vi "ResonanceScanner_V2.vi"() -> ()   [LabVIEW 2012]
uses:
  <vilib>/Platform/TimedLoop/XDataNode/timing_clust.ctl
  <vilib>/Platform/TimedLoop/XDataNode/nitl_modes.ctl
  <vilib>/Platform/TimedLoop/XDataNode/wakeup.ctl
  <vilib>/rvi/eio/common/nirviEmuTemplateMethod_errors.vi
  <vilib>/rvi/FIFO/Fifo_Resource/nirvififoEmulationSetSize.vi
  <vilib>/rvi/DataTransferAndStorage/Container/Common/niFpgaContainerGetUniqueNameForEmu.vi
  <vilib>/rvi/Emulation/niFpgaSctlEmulationRegisterWithScheduler.vi
  <vilib>/rvi/errors/niFpgaSetErrorForExecOnDevCompSimple.vi
  <vilib>/rvi/eio/common/nirviEmuReportErrorAndStop.vi
  <vilib>/rvi/Emulation/niFpgaSctlEmulationFifoFullMgr.vi
  <vilib>/rvi/Emulation/niFpgaSctlEmulationResourceMgr.vi
  <vilib>/rvi/Emulation/niFpgaSctlEmulationScheduler.vi
  <vilib>/rvi/interface/RandomDataEmulation/nirviRandomDataFPGAFIFO.vi
  <vilib>/rvi/interface/RandomDataEmulation/niFpgaRandomDataHandleErrors.vi
  <vilib>/rvi/Emulation/niFpgaSctlEmulationGlobalWrite.vi
  <vilib>/Platform/TimedLoop/XDataNode/XDataNode.xnode
  <vilib>/eio/EIONode/EIONode.xnode
  <vilib>/rvi/DataTransferAndStorage/Container/XNode/niFpgaContainer.xnode
  <vilib>/rvi/FIFO/Fifo_Resource/nirvififoEmulationClear.vi
  <vilib>/rvi/FIFO/Fifo_Resource/nirvififoEmulationWrite.vi
  <vilib>/rvi/FIFO/Fifo_Resource/nirvififoEmulationRead.vi
  <vilib>/rvi/interface/RandomDataEmulation/nirviRandomDataFpgaReadWriteTemplate.vi
  <vilib>/Platform/TimedLoop/XDataNode/XDNodeRunTimeDep.lvlib
panel:
  in  "Back delay":u16=10000
  in  "Forth delay":u16=10000
  in  "Baselinex8 Ch2":u16
  in  "Baselinex8 Ch1":u16
  in  "Clear Interloop FIFO":bool
  out "InterloopFIFO Timeout":bool
  out "ToHostCh2FIFO Overflow":bool
  out "ToHostCh1FIFO Overflow":bool
  out "Pixel counter":u32
  in  "Wait for trigger":bool
  in  "Acquire":bool
  in  "Acquire continuously":bool=TRUE
  in  "Requested pixels":u32=100000
  out "InterloopFIFO Overflow":bool
  out "Acquiring":bool
  in  "Samples per pixel":u32=10000 caption="Samples per pixel Acq"
  in  "Samples per line":u32=10000 caption="Samples per pixel Acq"
  out "Configured?":bool
  # "5751 IO module configuration"
  # "Resonance scanner V2"
  # "Acquisition control"
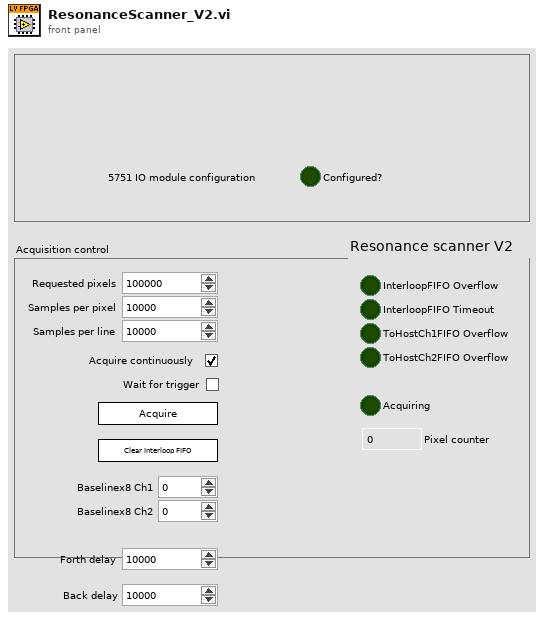
[diagram p1: front panel]
types:
  T1 = typedef "XDNodeRunTimeDep.lvlib/timing_clust.ctl" = cluster{"Expected End [f-1]":u64, "Actual End [f-1]":u64, "Finished Late? [f-1]":bool, "Expected End [i-1]":u64, "Actual End [i-1]":u64, "Finished Late? [i-1]":bool, "Expected Start [i]":u64, "Actual Start [i]":u64, "Expected Start [f]":u64, "Actual Start [f]":u64, "Source Name":string, "Structure Name":string, "Period":i64, "Deadline":i64, "Offset":i64, "Start":i64, "Priority":i32, "Timeout":i32, "Mode":T2, "Wakeup Reason":T3, "Error":errorcluster, "Source Type":string, "Secondary Source Type":string, "Global End Time":u64, "Global Start Time":u64, "Frame Duration":u64, "Iteration Duration":u64, "Assigned CPU":i32, "I/O Scan Engine Mode":u32}
  T2 = typedef "XDNodeRunTimeDep.lvlib/nitl_modes.ctl" = enum32{"No Change", "Process missed periods, maintain original phase", "Discard missed periods, maintain original phase", "Process missed periods, ignore original phase", "Discard missed periods, ignore original phase"}
  T3 = typedef "XDNodeRunTimeDep.lvlib/wakeup.ctl" = enum32{"Normal", "Aborted", "Asynchronous wakeup", "Timing source error", "Timed loop error", "Timeout"}
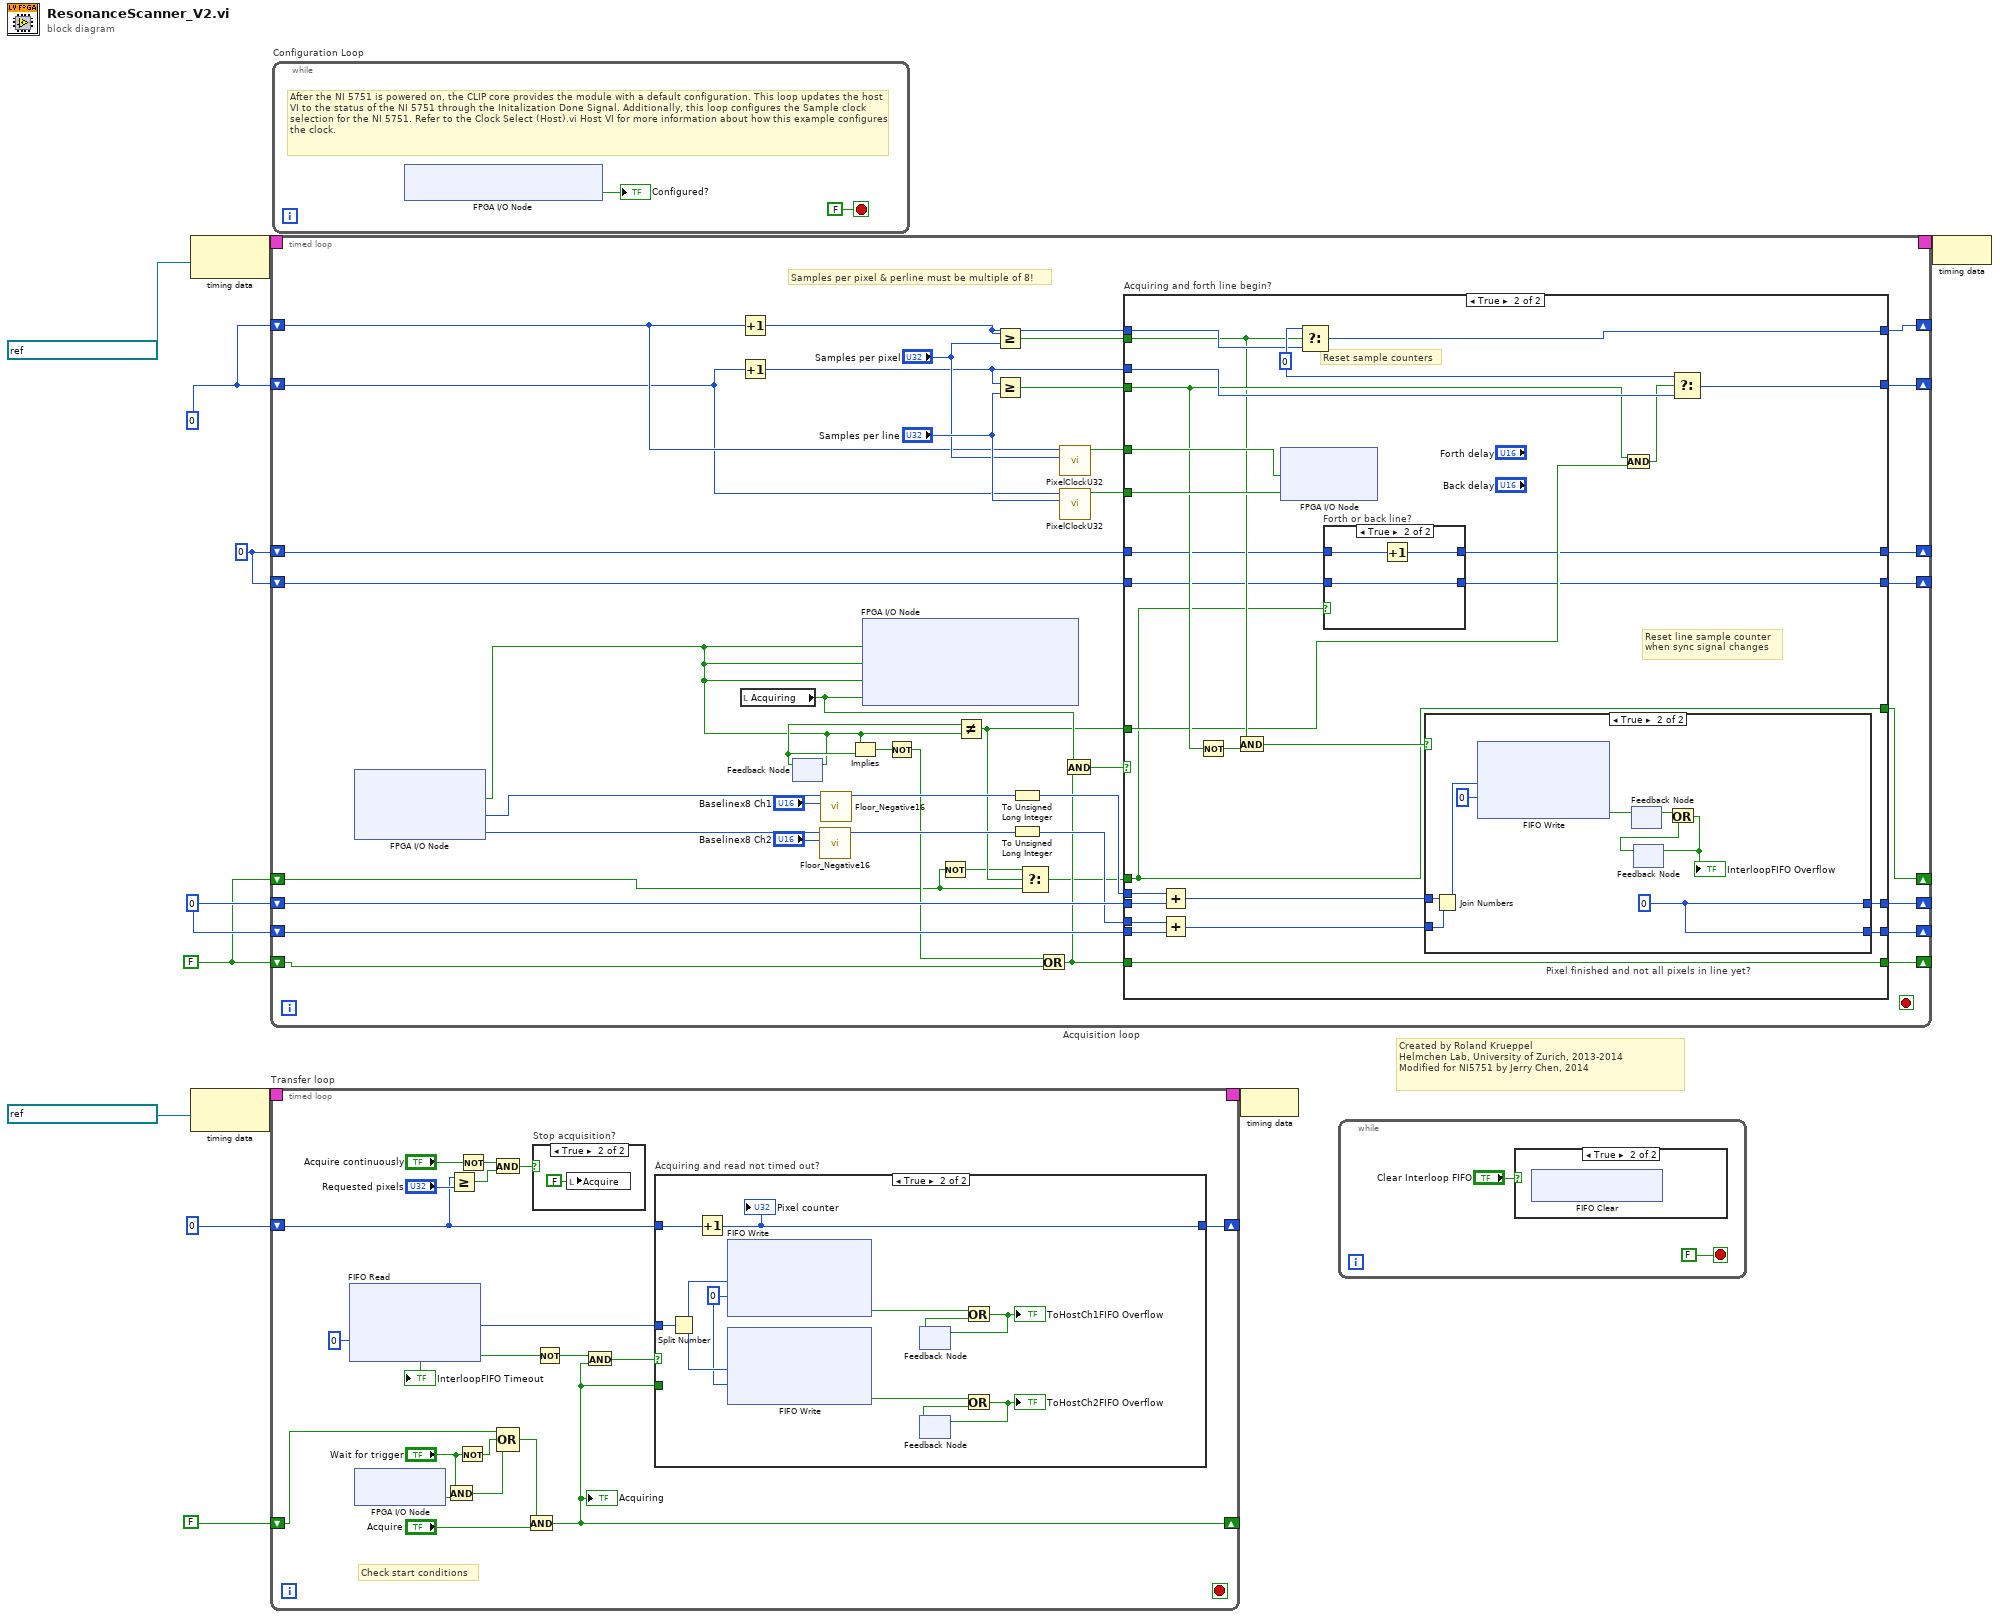
[diagram p0: block diagram]
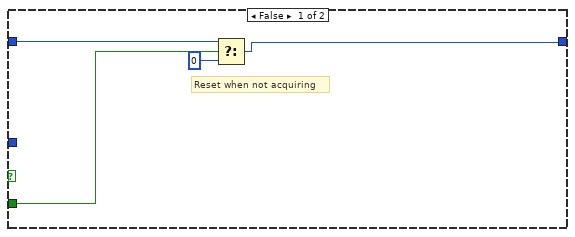
[diagram p4: hidden frame]
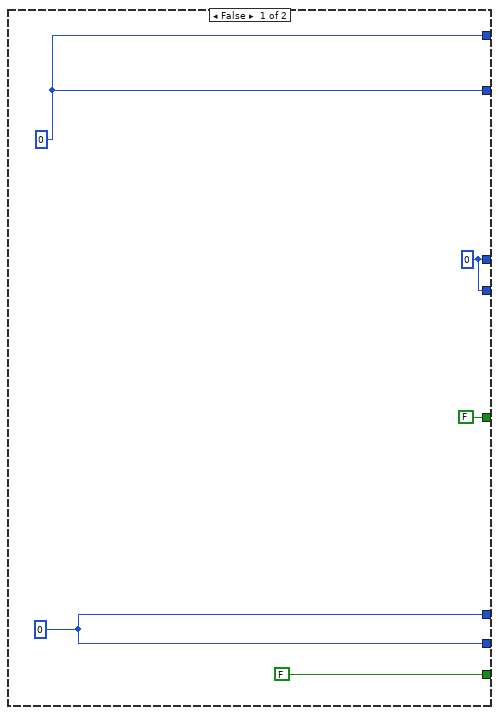
[diagram p5: hidden frame]
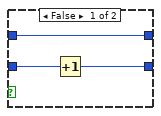
[diagram p6: hidden frame]
diagram:
  w2 = u16 0
  w1 = FALSE
  w9 = u32 0
  w10 = u32 0 ("t")
  # "Created by Roland Krueppel\nHelmchen Lab, University of Zurich, 2013-2014\nModified for NI5751 by Jerry Chen, 2014"
  n1 = node-c288(refnum<k21> "40 MHz Onboard Clock" ("Source Name")) -> (w12:T1)
  n2 = node-c288(refnum<k21> "40 MHz Onboard Clock" ("Source Name")) -> (w8:T1)
  n3 = timed-loop "Acquisition loop" {
    timing: w12 -> [_]
    timing-out: [_] -> w11
    shift-right: [w53] -> _
    shift-left: w10 -> [w34]
    shift-right: [w54] -> _
    shift-left: w10 -> [w36]
    shift-right: [w50] -> _
    shift-left: w9 -> [w52]
    shift-right: [w49] -> _
    shift-left: w9 -> [w51]
    shift-right: [w29] -> _
    shift-left: w1 -> [w28]
    shift-right: [w14] -> _
    shift-left: w2 -> [w21]
    shift-right: [w13] -> _
    shift-left: w2 -> [w20]
    shift-right: [w15] -> _
    shift-left: w1 -> [w17]
    stop <- _ stop-if-true
    # "Samples per pixel & perline must be multiple of 8!"
    n4 = xnode "FPGA I/O Node"() -> ("IO Module\\DI 0"=w22:bool, "IO Module\\AI A0"=w24:i16, "IO Module\\AI A2"=w23:i16)  [unwired: 3 in, 3 out]
    n5 = Increment(x=w36) -> (x+1=w35:u32)
    n6 = Increment(x=w34) -> (x+1=w33:u32)
    n7 = local read "Acquiring"() -> (w27:bool)
    n8 = feedback #1() -> (w32:bool)  [unwired: 1 in]
    n9 = feedback-in #1(w22) -> ()
    n10 = call "Floor_Negative16.vi"("Baseline U16"="Baselinex8 Ch2", "Input Value"=w23) -> ("Output Value"=w41:u16)  [unwired: 9 in]
    n11 = call "Floor_Negative16.vi"("Baseline U16"="Baselinex8 Ch1", "Input Value"=w24) -> ("Output Value"=w42:u16)  [unwired: 9 in]
    n12 = Implies(1:w32, 2:w22) -> (0:w31:bool)
    n13 = xnode "FPGA I/O Node"("IO Module\\D0 2"=w22, "IO Module\\D0 3"=w22, "IO Module\\D0 4"=w22, "IO Module\\Digital Output Enable"=w27) -> ()  [unwired: 4 in, 4 out]
    n14 = Not(x=w31) -> (.not. x?=w30:bool)
    n15 = Not(x=w17) -> (.not. x?=w18:bool)
    n16 = Not Equal?(x=w32, y=w22) -> (x != y?=w19:bool)
    n17 = Greater Or Equal?(x=w35, y="Samples per pixel") -> (x >= y?=w44:bool)
    n18 = Greater Or Equal?(x=w33, y="Samples per line") -> (x >= y?=w43:bool)
    n19 = To Unsigned Long Integer(number=w42) -> (unsigned 32bit integer=w38:u32)
    n20 = To Unsigned Long Integer(number=w41) -> (unsigned 32bit integer=w37:u32)
    n21 = Select(t=w18, s=w19, f=w17) -> (s? t:f=w16:bool)
    n22 = Or(x=w30, y=w28) -> (x .or. y?=w26:bool)
    n23 = call "PixelClockU32.vi"("Samples per pixel"="Samples per pixel", "Sample counter"=w36) -> ("Pixel clock"=w46:bool)  [unwired: 9 in]
    n24 = call "PixelClockU32.vi"("Samples per pixel"="Samples per line", "Sample counter"=w34) -> ("Pixel clock"=w45:bool)  [unwired: 9 in]
    n25 = And(x=w27, y=w26) -> (x .and. y?=w25:bool)
    n26 = case "Acquiring and forth line begin?" shown="True" w25 {
      tunnel: [w59 w85] -> w54
      tunnel: [w59 w84] -> w53
      tunnel: w38 -> [_ w82]
      tunnel: w52 -> [_ w83]
      tunnel: w51 -> [_ w81]
      tunnel: w37 -> [_ w80]
      tunnel: [w58 w77] -> w50
      tunnel: [w58 w76] -> w49
      tunnel: w44 -> [_ w67]
      tunnel: w43 -> [_ w68]
      tunnel: w35 -> [_ w75]
      tunnel: w33 -> [_ w74]
      tunnel: w46 -> [_ w73]
      tunnel: w45 -> [_ w72]
      tunnel: w19 -> [_ w66]
      tunnel: w26 -> [_ w65]
      tunnel: [FALSE w65] -> w29
      tunnel: w21 -> [_ w64]
      tunnel: w20 -> [_ w63]
      tunnel: w16 -> [_ w62]
      tunnel: [FALSE w62] -> w15
      tunnel: [w55 w61] -> w14
      tunnel: [w55 w60] -> w13
      frame False {
        w55 = u16 0
        w58 = u32 0
        w59 = u16 0 ("t")
      }
      frame True {
        w86 = u32 0 ("t")
        # "Reset line sample counter\nwhen sync signal changes"
        # "Reset sample counters"
        n27 = Add(x=w82, y=w83) -> (x+y=w78:u32)
        n28 = Add(x=w80, y=w81) -> (x+y=w79:u32)
        n29 = Not(x=w68) -> (.not. x?=w71:bool)
        n30 = And(x=w67, y=w71) -> (x .and. y?=w70:bool)
        n31 = xnode "FPGA I/O Node"("PixelClock"=w73, "LineClock"=w72) -> ()  [unwired: 2 in, 2 out]
        n32 = Select(t=w86, s=w67, f=w75) -> (s? t:f=w85:u32)
        n33 = case "Forth or back line?" shown="True" w62 {
          tunnel: w64 -> [w87 w92]
          tunnel: w63 -> [w89 w90]
          tunnel: [w87 w91] -> w61
          tunnel: [w88 w90] -> w60
          frame False {
            n34 = Increment(x=w89) -> (x+1=w88:u16)
          }
          frame True {
            n35 = Increment(x=w92) -> (x+1=w91:u16)
          }
        }
        n36 = case "Pixel finished and not all pixels in line yet?" shown="True" w70 {
          tunnel: w79 -> [w93 w96]
          tunnel: w78 -> [w94 w97]
          tunnel: [w94 w100] -> w77
          tunnel: [w93 w100] -> w76
          frame False {
          }
          frame True {
            w100 = u32 0
            n37 = Join Numbers(hi=w97, lo=w96) -> ((hi.lo)=w95:u64)
            n38 = xnode ("FIFO Write")("Element"=w95, "Timeout"=0) -> ("Timed Out?"=w98:bool)  [unwired: 1 in, 1 out]
            n39 = feedback-in #2(w98) -> ()
            n40 = feedback #2() -> (w99:bool)  [unwired: 1 in]
            n41 = feedback #3() -> (w101:bool)  [unwired: 1 in]
            n42 = Or(x=w99, y=w101) -> (x .or. y?=w102:bool)
            "InterloopFIFO Overflow" <- w102
            n43 = feedback-in #3(w102) -> ()
          }
        }
        n44 = And(x=w68, y=w66) -> (x .and. y?=w69:bool)
        n45 = Select(t=w86, s=w69, f=w74) -> (s? t:f=w84:u32)
      }
    }
  }
  n46 = timed-loop "Transfer loop" {
    timing: w8 -> [_]
    timing-out: [_] -> w7
    shift-right: [w108] -> _
    shift-left: u32 0 -> [w109]
    shift-right: [w107] -> _
    shift-left: FALSE -> [w115]
    stop <- _ stop-if-true
    # "Check start conditions"
    n47 = xnode ("FIFO Read")("Timeout"=0) -> ("Element"=w110:u64, "Timed Out?"=w114:bool)  [unwired: 1 in, 1 out]
    "InterloopFIFO Timeout" <- w114
    n48 = xnode "FPGA I/O Node"() -> ("TriggerIn"=w120:bool)  [unwired: 1 in, 1 out]
    n49 = And(x="Wait for trigger", y=w120) -> (x .and. y?=w117:bool)
    n50 = Greater Or Equal?(x=w109, y="Requested pixels") -> (x >= y?=w122:bool)
    n51 = Not(x="Wait for trigger") -> (.not. x?=w118:bool)
    n52 = Not(x="Acquire continuously") -> (.not. x?=w123:bool)
    n53 = And(x=w123, y=w122) -> (x .and. y?=w112:bool)
    n54 = Compound Arithmetic op=OR(w115, w118, w117) -> (w116:bool)
    n55 = And(x=w116, y="Acquire") -> (x .and. y?=w107:bool)
    "Acquiring" <- w107
    n56 = case "Stop acquisition?" shown="True" w112 {
      frame False {
      }
      frame True {
        n57 = local write "Acquire"(FALSE ("Acquire")) -> ()
      }
    }
    n58 = Not(x=w114) -> (.not. x?=w113:bool)
    n59 = And(x=w113, y=w107) -> (x .and. y?=w111:bool)
    n60 = case "Acquiring and read not timed out?" shown="True" w111 {
      tunnel: w110 -> [_ w142]
      tunnel: w109 -> [w129 w138]
      tunnel: [w128 w137] -> w108
      tunnel: w107 -> [w130 _]
      frame False {
        # "Reset when not acquiring"
        n61 = Select(t=w129, s=w130, f=u32 0) -> (s? t:f=w128:u32)
      }
      frame True {
        w139 = 0 ("Timeout")
        n62 = Split Number(x=w142) -> (hi(x)=w141:u32, lo(x)=w140:u32)
        n63 = Increment(x=w138) -> (x+1=w137:u32)
        "Pixel counter" <- w137
        n64 = xnode ("FIFO Write")("Element"=w141, "Timeout"=w139) -> ("Timed Out?"=w135:bool)  [unwired: 1 in, 1 out]
        n65 = xnode ("FIFO Write")("Element"=w140, "Timeout"=w139) -> ("Timed Out?"=w132:bool)  [unwired: 1 in, 1 out]
        n66 = feedback #4() -> (w134:bool)  [unwired: 1 in]
        n67 = feedback #5() -> (w131:bool)  [unwired: 1 in]
        n68 = Or(x=w135, y=w134) -> (x .or. y?=w136:bool)
        "ToHostCh1FIFO Overflow" <- w136
        n69 = feedback-in #4(w136) -> ()
        n70 = Or(x=w132, y=w131) -> (x .or. y?=w133:bool)
        "ToHostCh2FIFO Overflow" <- w133
        n71 = feedback-in #5(w133) -> ()
      }
    }
  }
  n72 = while "Configuration Loop" {
    stop <- FALSE stop-if-true
    # "After the NI 5751 is powered on, the CLIP core provides the module with a default configuration. This loop updates the host VI to the status of the NI 5751 through the Initalization Done Signal. Additionally, this loop configures the Sample clock selection for the NI 5751. Refer to the Clock Select (Host).vi Host VI for more information about how this example configures the clock."
    n73 = xnode "FPGA I/O Node"() -> ("IO Module\\Initialization Done"=→"Configured?":bool)  [unwired: 1 in, 1 out]
  }
  n74 = node-c288(w7) -> ()
  n75 = while {
    stop <- FALSE stop-if-true
    n76 = case shown="True" "Clear Interloop FIFO" {
      frame False {
      }
      frame True {
        n77 = xnode ("FIFO Clear")() -> ()  [unwired: 1 in, 1 out]
      }
    }
  }
  n78 = node-c288(w11) -> ()
